vi "TEST - KICKER BUTTON PRESS.vi"(8 "error in (no error)":errorcluster, 10 "Cluster of JOYSTICK and KICKER ref info":T8, 11 "refnum name":string) -> (0 "error out":errorcluster)   [LabVIEW 2020]
uses:
  <vilib>/Rock Robotics/WPI/Joystick/WPI_JoystickDevRef.ctl
  <vilib>/Rock Robotics/WPI/Joystick/WPI_JoystickDeviceEnum.ctl
  <vilib>/Rock Robotics/WPI/MotorControl/WPI_MotorControlDeviceRef.ctl
  <vilib>/Rock Robotics/WPI/MotorControl/WPI_MotorControlType.ctl
  <vilib>/Rock Robotics/SystemInterfaces/DIO/FPGA_DIOPWMChannel.ctl
  <vilib>/Rock Robotics/WPI/PWM/WPI_PWMDeadband.ctl
  <vilib>/Rock Robotics/SystemInterfaces/DIO/FPGA_DIOChannel.ctl
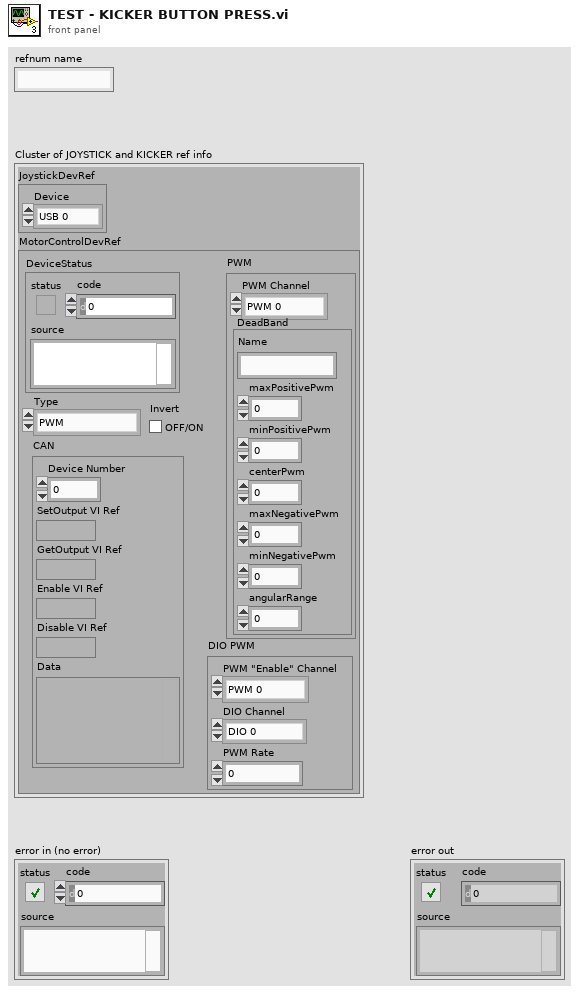
[diagram p1: front panel]
types:
  T1 = typedef "WPI_JoystickDevRef.ctl" = cluster{"Device":T2}
  T2 = typedef "WPI_JoystickDeviceEnum.ctl" = enum16{"USB 0", "USB 1", "USB 2", "USB 3", "USB 4", "USB 5"}
  T3 = typedef "WPI_MotorControlDeviceRef.ctl" = cluster{"DeviceStatus":errorcluster, "Type":T4, "PWM":cluster{"PWM Channel":T5, "DeadBand":T6}, "CAN":cluster{"Device Number":u8, "SetOutput VI Ref":variant, "GetOutput VI Ref":variant, "Enable VI Ref":variant, "Disable VI Ref":variant, "Data":variant}, "Invert":bool, "DIO PWM":cluster{"PWM \"Enable\" Channel":T5, "DIOChannel":T7, "PWM Rate":dbl}}
  T4 = typedef "WPI_MotorControlType.ctl" = enum16{"PWM", "CAN", "DIO PWM"}
  T5 = typedef "FPGA_DIOPWMChannel.ctl" = enum8{"PWM 0", "PWM 1", "PWM 2", "PWM 3", "PWM 4", "PWM 5", "PWM 6", "PWM 7", "PWM 8", "PWM 9", "PWM MXP 0", "PWM MXP 1", "PWM MXP 2", "PWM MXP 3", "PWM MXP 4", "PWM MXP 5", "PWM MXP 6", "PWM MXP 7", "PWM MXP 8", "PWM MXP 9", "Invalid"}
  T6 = typedef "WPI_PWMDeadband.ctl" = cluster{"Name":string, "maxPositivePwm":i32, "minPositivePwm":i32, "centerPwm":i32, "maxNegativePwm":i32, "minNegativePwm":i32, "angularRange":u16}
  T7 = typedef "FPGA_DIOChannel.ctl" = enum8{"DIO 0", "DIO 1", "DIO 2", "DIO 3", "DIO 4", "DIO 5", "DIO 6", "DIO 7", "DIO 8", "DIO 9", "DIO MXP 0", "DIO MXP 1", "DIO MXP 2", "DIO MXP 3", "DIO MXP 4", "DIO MXP 5", "DIO MXP 6", "DIO MXP 7", "DIO MXP 8", "DIO MXP 9", "DIO MXP 10", "DIO MXP 11", "DIO MXP 12", "DIO MXP 13", "DIO MXP 14", "DIO MXP 15", "SPI Port CS1", "SPI Port CS2", "SPI Port CS3", "SPI Port MISO", "SPI Port MOSI", "Invalid"}
  T8 = cluster{"JoystickDevRef":T1, "MotorControlDevRef":T3}
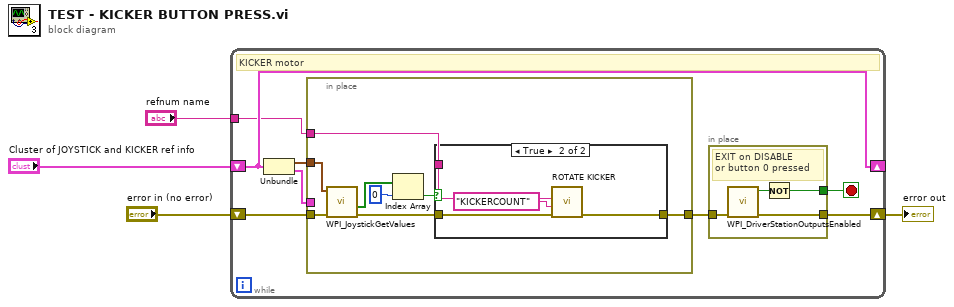
[diagram p0: block diagram]
diagram:
  n1 = while {
    shift-right: [w12] -> _
    shift-left: "Cluster of JOYSTICK and KICKER ref info" -> [w12]
    tunnel: "refnum name" -> [w7]
    shift-right: [w6] -> w1
    shift-left: "error in (no error)" -> [w5]
    stop <- w9 stop-if-true
    # "KICKER motor"
    n2 = Unbundle(w12) -> ("JoystickDevRef"=w11:T1, "MotorControlDevRef"=w10:T3)
    n3 = in-place {
      in-place-border: w11 -> [w20]
      in-place-border: w10 -> [_]
      in-place-border: [w15] -> w8
      in-place-border: w5 -> [w17]
      in-place-border: w7 -> [w13]
      n4 = call <vilib>:"WPI_JoystickGetValues.vi"("error in (no error)"=w17, "JoystickDevRef"=w20) -> ("error out"=w14:errorcluster, "Buttons"=w19:bool[])  [unwired: 5 in, 3 out]
      n5 = Index Array(array=w19, index=0) -> (element=w16:bool)
      n6 = case shown="True" w16 {
        tunnel: [w21 w25] -> w15
        tunnel: w14 -> [w21 w23]
        tunnel: w13 -> [_ w22]
        frame False {
        }
        frame True {
          n7 = call "ROTATE KICKER.vi"("error in (no error)"=w23, "RefName COUNT"="KICKERCOUNT", "RefName KICKER"=w22) -> ("error out"=w25:errorcluster)  [unwired: 8 in]
        }
      }
    }
    n8 = in-place {
      in-place-border: [w26] -> w9
      in-place-border: w8 -> [w28]
      in-place-border: [w27] -> w6
      # "EXIT on DISABLE\nor button 0 pressed"
      n9 = call <vilib>:"WPI_DriverStationOutputsEnabled.vi"("error in"=w28) -> ("error out"=w27:errorcluster, "OutputsEnabled?"=w29:bool)  [unwired: 9 in]
      n10 = Not(x=w29) -> (.not. x?=w26:bool)
    }
  }
  "error out" <- w1
